vi "Read Pulse Configuration.vi"(8 "error in (no error)":errorcluster, 11 "DAQmx DAQmx Lockin Digitizer Driver in":refnum<class "DAQmx Lockin Digitizer Driver.lvclass">) -> (0 "error out":errorcluster, 2 "Configuration":T1={"Post-trigger delay"=0.01, "Post-trigger duration"=0.1, "Rate"=1000000.0, "Ranges"=[10.0], "Re-name channels"=[], "Active channels"="0:1", "External clock"=FALSE} {"Rate" format="%#_8pHz"; "Post-trigger duration" format="%#_6ps"; "Post-trigger delay" format="%#_6ps"; "Ranges" format="%#_6pV"}, 3 "DAQmx DAQmx Lockin Digitizer Driver in":refnum<class "DAQmx Lockin Digitizer Driver.lvclass">)   [LabVIEW 2021, in "DAQmx Lockin Digitizer Driver.lvclass"]
uses:
  DAQmx Lockin Digitizer Driver.lvclass
  DAQmx Lockin Digitizer Driver.lvclass/DAQmx Lockin Digitizer Driver.ctl
  Instruments/Pulse Driver/Pusle Driver Configuration.ctl
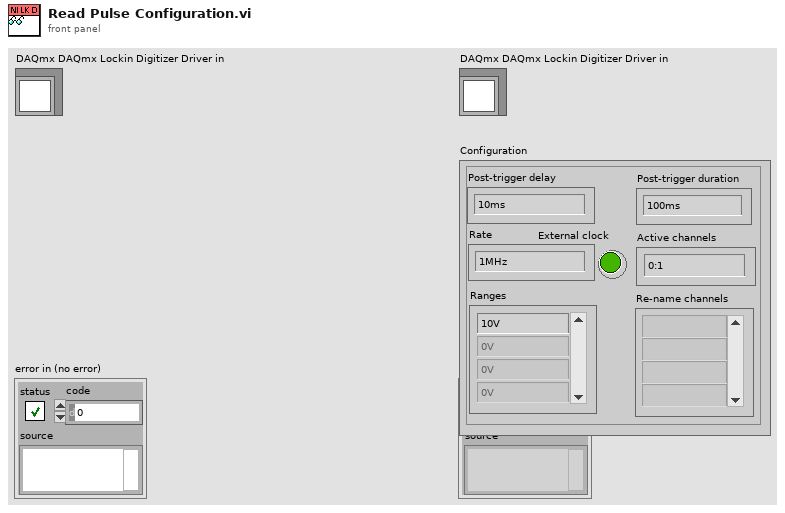
[diagram p1: front panel]
types:
  T1 = typedef "Pusle Driver Configuration.ctl" = cluster{"Post-trigger delay":dbl, "Post-trigger duration":dbl, "Rate":dbl, "Ranges":dbl[], "Re-name channels":string[], "Active channels":string, "External clock":bool}
  T2 = typedef "Lockin Digitizer Configuration.ctl" = cluster{"Post-trigger delay":dbl, "Post-trigger duration":dbl, "Rate":dbl, "Ranges":dbl[], "Re-name channels":string[], "Active channels":string, "External\nclock":bool, "Frequencies":dbl[], "Time\nconstant":dbl, "Output \namplitudes":dbl[], "Input\nchannles":string[]}
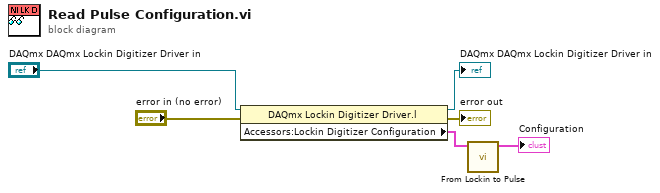
[diagram p0: block diagram]
diagram:
  n1 = property class="DAQmx Lockin Digitizer Driver.l"(reference="DAQmx DAQmx Lockin Digitizer Driver in", error in="error in (no error)") -> (reference out=→"DAQmx DAQmx Lockin Digitizer Driver in":refnum<class "DAQmx Lockin Digitizer Driver.lvclass">, error out=→"error out":errorcluster, "Accessors:Lockin Digitizer Configuration"=w6:T2)
  n2 = call "From Lockin to Pulse .vi"("Lockin Configuration in"=w6) -> ("Pulse  Configuration out"=→"Configuration":T1)  [unwired: 10 in]
